vi "Auto Gears.vi"(9 "Low Gear Speed":dbl, 10 "Left Encoder Velocity":dbl, 11 "Right Encoder Velocity":dbl) -> ()   [LabVIEW 2016]
uses:
  Framework/Robot Global Data.vi
panel:
  in  "x":bool
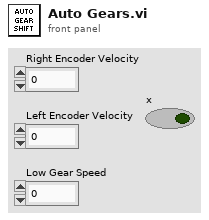
[diagram p1: front panel]
types:
  T1 = typedef "WPI_DriverStationRobotMode2.ctl" = enum16{"Autonomous Disabled", "Autonomous Enabled", "Teleop Disabled", "Teleop Enabled", "Disconnected", "Finish", "Test Disabled", "Test Enabled", "Emergency Stopped"}
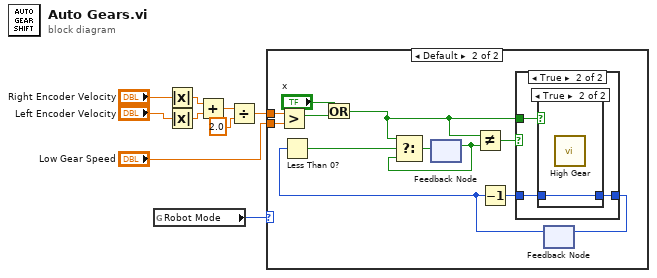
[diagram p0: block diagram]
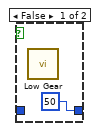
[diagram p4: hidden frame]
diagram:
  n1 = global read "Robot Global Data.vi" "Robot Mode"() -> (w9:T1)
  n2 = Absolute Value(x="Right Encoder Velocity") -> (abs(x)=w4:dbl)
  n3 = Absolute Value(x="Left Encoder Velocity") -> (abs(x)=w3:dbl)
  n4 = Add(x=w4, y=w3) -> (x+y=w5:dbl)
  n5 = Divide(x=w5, y=2.0) -> (x/y=w7:dbl)
  n6 = case shown="Default" w9 {
    tunnel: w7 -> [_ w21]
    tunnel: "Low Gear Speed" -> [_ w20]
    frame "Autonomous Enabled" {
    }
    frame Default {
      n7 = Greater?(x=w21, y=w20) -> (0:w12:bool)
      n8 = Or(x="x", y=w12) -> (x .or. y?=w11:bool)
      n9 = feedback #1() -> (w13:bool)  [unwired: 1 in]
      n10 = Not Equal?(x=w11, y=w13) -> (x != y?=w19:bool)
      n11 = feedback #2() -> (w15:i32)  [unwired: 1 in]
      n12 = Less Than 0?(x=w15) -> (x < 0?=w14:bool)
      n13 = Select(t=w11, s=w14, f=w13) -> (s? t:f=w16:bool)
      n14 = feedback-in #1(w16) -> ()
      n15 = Decrement(x=w15) -> (x-1=w17:i32)
      n16 = case shown="True" w19 {
        tunnel: w11 -> [_ w25]
        tunnel: [w22 w24] -> w18
        tunnel: w17 -> [w22 w23]
        frame False {
        }
        frame True {
          n17 = case shown="True" w25 {
            tunnel: [50 w27] -> w24
            tunnel: w23 -> [_ w27]
            frame False {
              n18 = call "Low Gear.vi"() -> ()  [unwired: 12 in]
            }
            frame True {
              n19 = call "High Gear.vi"() -> ()  [unwired: 12 in]
            }
          }
        }
      }
      n20 = feedback-in #2(w18) -> ()
    }
  }
